vi "nndirectcontrol.vi"() -> ()   [LabVIEW 2017]
doc: "The Clap Sensor sample project implements a clap sensor that detects claps and displays the intensity of the claps by using the onboard LEDs of myRIO."
uses:
  <vilib>/myRIO/Instrument Drivers/Onboard IO/AI/typedefs/AI Reference.ctl
  <vilib>/myRIO/Common/Instrument Driver Framework/Utilities/typedefs/myRIO Generic Hardware Reference.ctl
  <vilib>/myRIO/Common/Instrument Driver Framework/Utilities/typedefs/Hardware Version Enum.ctl
  <vilib>/myRIO/Common/Instrument Driver Framework/Utilities/typedefs/myRIO v1.0 Reference.ctl
  <vilib>/myRIO/Common/Instrument Driver Framework/Utilities/typedefs/Generic FPGA Reference.ctl
  <vilib>/myRIO/Common/Instrument Driver Framework/myRIO v1.0/AI/typedefs/AI Channels List.ctl
  <vilib>/myRIO/Common/Instrument Driver Framework/myRIO v1.0/AI/typedefs/AI Channels Enum.ctl
  <vilib>/myRIO/Common/Instrument Driver Framework/Utilities/typedefs/Analog Scaling Constants List.ctl
  <vilib>/myRIO/Common/Instrument Driver Framework/Utilities/typedefs/Analog Scaling Constants.ctl
  <vilib>/userdefined/High Color/nirio_resource_hc.ctl
  <vilib>/myRIO/Instrument Drivers/Onboard IO/PWM/typedefs/PWM Reference.ctl
  <vilib>/myRIO/Common/Instrument Driver Framework/myRIO v1.0/PWM/typedefs/PWM Channels Enum.ctl
  <vilib>/myRIO/Instrument Drivers/Onboard IO/PWM/typedefs/PWM Configuration.ctl
  <vilib>/myRIO/Common/Instrument Driver Framework/Utilities/vis/Is FPGA Ref Available.vi
  <vilib>/myRIO/Common/Instrument Driver Framework/myRIO v1.0/AI/vis/myRIO v1.1 Open AI.vi
  <vilib>/myRIO/Instrument Drivers/Onboard IO/AI/vis/Read.vi
  <vilib>/myRIO/Common/Instrument Driver Framework/myRIO v1.0/PWM/vis/myRIO v1.1 Open PWM.vi
  <vilib>/myRIO/Instrument Drivers/Onboard IO/PWM/vis/Set Duty Cycle and Frequency.vi
  <vilib>/myRIO/Common/Instrument Driver Framework/Utilities/vis/Validate Channels.vi
  <vilib>/myRIO/Common/Instrument Driver Framework/myRIO v1.0/AI/vis/myRIO v1.0 Reserve AI.vi
  <vilib>/myRIO/Common/Instrument Driver Framework/myRIO v1.0/PWM/vis/myRIO v1.0 Reserve PWM.vi
  <vilib>/myRIO/Common/Instrument Driver Framework/myRIO v1.0/UART/vis/myRIO v1.0 Close UART.vi
  <vilib>/myRIO/Common/Instrument Driver Framework/myRIO v1.0/AI/vis/myRIO v1.0 Build MUX Configuration AI.vi
  <vilib>/myRIO/Common/Instrument Driver Framework/myRIO v1.0/Resource Manager/vis/myRIO v1.0 Reserve Channel List.vi
  <vilib>/myRIO/Common/Instrument Driver Framework/myRIO v1.0/PWM/vis/myRIO v1.0 Build MUX Configuration PWM.vi
  <vilib>/myRIO/Common/Instrument Driver Framework/myRIO v1.0/Resource Manager/vis/myRIO v1.0 Reserve Channel.vi
  <vilib>/myRIO/Common/Instrument Driver Framework/myRIO v1.0/Resource Manager/vis/myRIO v1.0 Unreserve Channel.vi
  <vilib>/myRIO/Common/Instrument Driver Framework/myRIO v1.0/Resource Manager/vis/myRIO v1.0 Create Configuration List.vi
  <vilib>/myRIO/Common/Instrument Driver Framework/myRIO v1.0/Resource Manager/vis/myRIO v1.0 Build Mutex Name.vi
  <vilib>/Utility/VariantDataType/GetNumericInfo.vi
  <vilib>/Utility/error.llb/Error Cluster From Error Code.vi
  <vilib>/myRIO/Common/Instrument Driver Framework/myRIO v1.0/myRIO v1.1 Open.vi
  <vilib>/myRIO/Common/Instrument Driver Framework/myRIO v1.0/AI/vis/myRIO v1.0 Get Scaling Constants AI.vi
  <vilib>/myRIO/Common/Instrument Driver Framework/Utilities/vis/IO Manager.vi
  <vilib>/myRIO/Common/Instrument Driver Framework/Utilities/vis/Configuration Manager.vi
  <vilib>/myRIO/Common/Instrument Driver Framework/myRIO v1.0/myRIO v1.0 Close.vi
  <vilib>/myRIO/Common/Instrument Driver Framework/myRIO v1.0/AI/vis/myRIO v1.0 Read AI.vi
  <vilib>/imath/engines/lvmath2/RunTimeEngine/IndexRead/NIMS M(S,S).vi
  <instcachedir>/0/NIMS M(S,S)_AC51E74150A542F7991B9634C66F3096.lvgen/NIMS M(S,S)_AC51E74150A542F7991B9634C66F3096_000.vi
  <vilib>/imathl/engines/lvmath/Functions/Error Handling/Create Error.vi
  <vilib>/imath/engines/lvmath2/RunTimeEngine/IndexReplace/NIMS V(S)=S.vi
  <instcachedir>/0/NIMS V(S)=S_3F4D177D41884A9C969E5FA0B22E4B28.lvgen/NIMS V(S)=S_3F4D177D41884A9C969E5FA0B22E4B28_000.vi
  <vilib>/imath/engines/lvmath2/RunTimeEngine/IndexRead/NIMS V(S).vi
  <instcachedir>/0/NIMS V(S)_0488751826AF41519A22953C041130DC.lvgen/NIMS V(S)_0488751826AF41519A22953C041130DC_000.vi
  <vilib>/imath/engines/lvmath2/RunTimeEngine/ErrorHandling/NIMS_Create Error From Enums.vi
  <vilib>/imath/engines/lvmath2/RunTimeEngine/IndexReplace/NIMS M(S,S)=S.vi
  <instcachedir>/0/NIMS M(S,S)=S_490F2BBDD0204024B81939EC402D9A55.lvgen/NIMS M(S,S)=S_490F2BBDD0204024B81939EC402D9A55_000.vi
  <vilib>/imath/engines/lvmath2/RunTimeEngine/NodeEndStatement/NIMS_NodeEndStatement_Output.vi
  <instcachedir>/0/NIMS_NodeEndStatement_Output_53EC0D466D134D7ABD903AC30B43404B.lvgen/NIMS_NodeEndStatement_Output_53EC0D466D134D7ABD903AC30B43404B_001.vi
  <instcachedir>/0/NIMS_NodeEndStatement_Output_53EC0D466D134D7ABD903AC30B43404B.lvgen/NIMS_NodeEndStatement_Output_53EC0D466D134D7ABD903AC30B43404B_005.vi
  <instcachedir>/0/NIMS_NodeEndStatement_Output_53EC0D466D134D7ABD903AC30B43404B.lvgen/NIMS_NodeEndStatement_Output_53EC0D466D134D7ABD903AC30B43404B_002.vi
  <vilib>/imath/engines/lvmath2/RunTimeEngine/ErrorHandling/NIMS_Finalize Error.vi
  <vilib>/myRIO/Common/Instrument Driver Framework/myRIO v1.0/Resource Manager/vis/myRIO v1.0 Configure IO.vi
  <vilib>/myRIO/Common/Instrument Driver Framework/myRIO v1.0/PWM/vis/myRIO v1.0 Write PWM.vi
  <vilib>/myRIO/Common/Instrument Driver Framework/Utilities/vis/FPGA Ref Manager.vi
  <vilib>/myRIO/Common/Instrument Driver Framework/myRIO v1.0/myRIO v1.0 Reset FPGA.vi
  <vilib>/myRIO/Common/Instrument Driver Framework/myRIO v1.0/IRQ/vis/myRIO v1.0 IRQ Info FGV.vi
  <vilib>/myRIO/Common/Instrument Driver Framework/myRIO v1.0/IRQ/vis/myRIO v1.0 Timer IRQ Info FGV.vi
  <vilib>/myRIO/Common/Instrument Driver Framework/myRIO v1.0/IRQ/vis/myRIO v1.0 ISR Agent.vi
  <vilib>/myRIO/Express VI/Onboard IO/AI/AI Express VI.xnode
  <vilib>/myRIO/Instrument Drivers/Onboard IO/AI/vis/myRIO AI Open.xnode
  <vilib>/myRIO/Express VI/Onboard IO/PWM/PWM Express VI.xnode
  <vilib>/myRIO/Instrument Drivers/Onboard IO/PWM/vis/myRIO PWM Open.xnode
  <vilib>/myRIO/Instrument Drivers/Utilities/Utilities.lvlib
  <vilib>/myRIO/Instrument Drivers/Onboard IO/AI/AI.lvlib
  <vilib>/myRIO/Instrument Drivers/Onboard IO/PWM/PWM.lvlib
panel:
  in  "step":dbl
  in  "delay":dbl
  in  "max":dbl
  in  "min":dbl
  in  "Staircase":bool
  in  "Sine Ampl.":dbl(slide) scale=0.0..0.5
  in  "Sine freq.":dbl(slide) scale=0.025..0.2
  out "Waveform Chart 2":dbl(graph)
  out "Waveform Chart":cluster{"pa":dbl, "Pdeseada":dbl}(graph)
  out "error [%]":dbl
  in  "PWM [Hz]":dbl=60.0 min=60.0 step=5.0
  out "e1":dbl
  out "eo":dbl
  in  "sample time":u32=20 min=20 step=5
  out "Potentiometer":dbl
  out "yk":dbl
  out "v":dbl[](array[numeric])
  out "w":dbl[][](array[numeric])
  in  "eta":dbl
  in  "Stop":bool
  in  "Pot. (Desired)":dbl=2.0 min=1.6 max=3.6 step=0.2
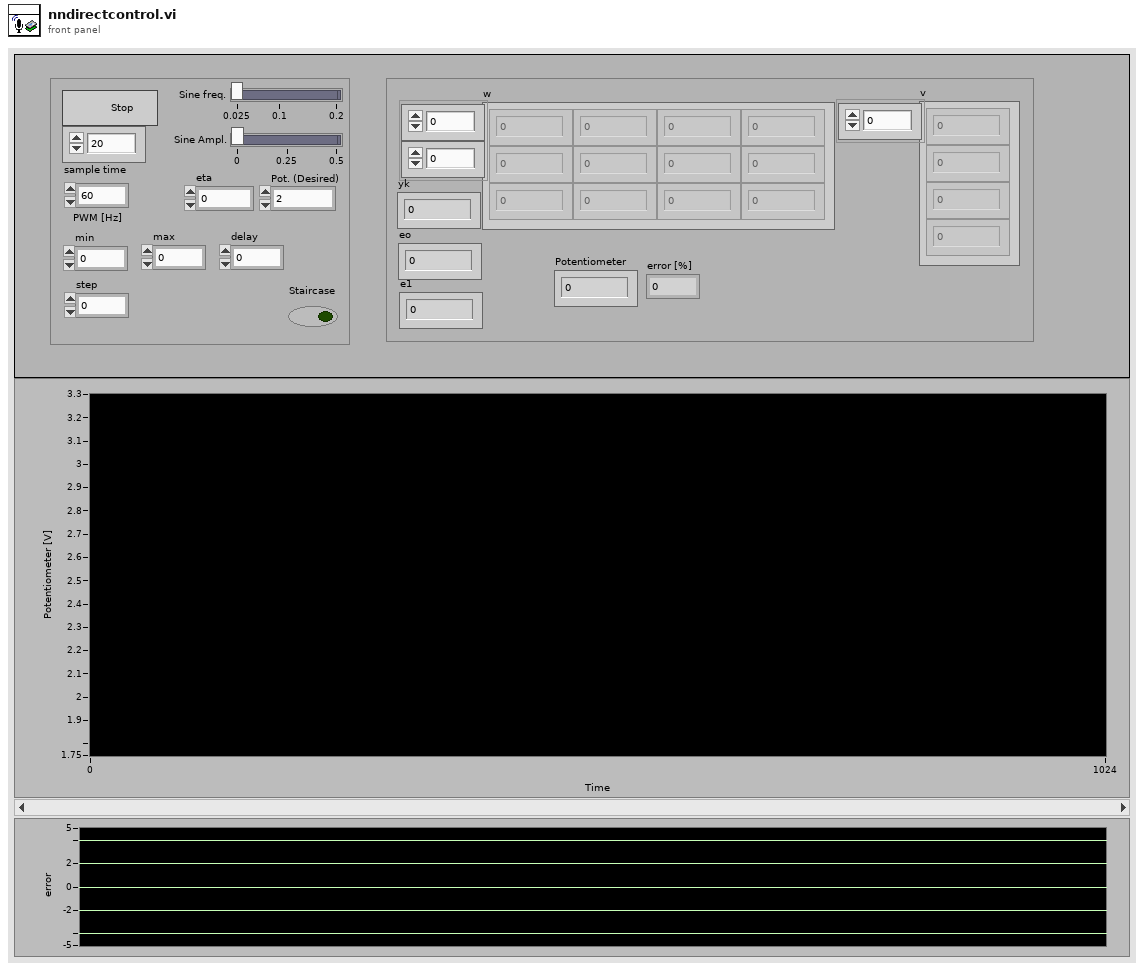
[diagram p1: front panel]
types:
  T1 = typedef "PWM.lvlib/PWM Reference.ctl" = cluster{"myRIO Reference":T2, "PWM Channels Enum":T6, "PWM Configuration":T7}
  T2 = typedef "myRIO Generic Hardware Reference.ctl" = cluster{"myRIO Model":T3, "myRIO Hardware Reference":T4}
  T3 = typedef "Hardware Version Enum.ctl" = enum16{"Unknown", "myRIO-1900", "myRIO-1950", "roboRIO", "NI ELVIS RIO CM"}
  T4 = typedef "myRIO v1.0 Reference.ctl" = cluster{"Generic FPGA Reference":T5, "Allow multiple opens":bool}
  T5 = typedef "Generic FPGA Reference.ctl" = refnum<k20>
  T6 = typedef "PWM Channels Enum.ctl" = enum16{"Not Connected", "C/PWM0", "C/PWM1", "A/PWM0", "A/PWM1", "A/PWM2", "B/PWM0", "B/PWM1", "B/PWM2", "PWM/PWM0", "PWM/PWM1", "PWM/PWM2", "PWM/PWM3", "PWM/PWM4", "PWM/PWM5", "PWM/PWM6", "PWM/PWM7", "PWM/PWM8", "PWM/PWM9"}
  T7 = typedef "PWM.lvlib/PWM Configuration.ctl" = cluster{"Frequency":dbl, "Duty Cycle":dbl}
  T8 = typedef "nirio_resource_hc.ctl" = tag
  T9 = typedef "AI.lvlib/AI Reference.ctl" = cluster{"myRIO Reference":T2, "AI Channels List":T10, "AI Scaling Constants List":T12}
  T10 = typedef "AI Channels List.ctl" = T11[]
  T11 = typedef "AI Channels Enum.ctl" = enum16{"Not Connected", "AudioIn/Left", "AudioIn/Right", "C/AI0", "C/AI1", "A/AI0", "A/AI1", "A/AI2", "A/AI3", "B/AI0", "B/AI1", "B/AI2", "B/AI3", "AI/AI0", "AI/AI1", "AI/AI2", "AI/AI3"}
  T12 = typedef "Analog Scaling Constants List.ctl" = T13[]
  T13 = typedef "Analog Scaling Constants.ctl" = cluster{"LSB Weight (Volts)":dbl, "Offset (Volts)":dbl, "Signed?":bool}
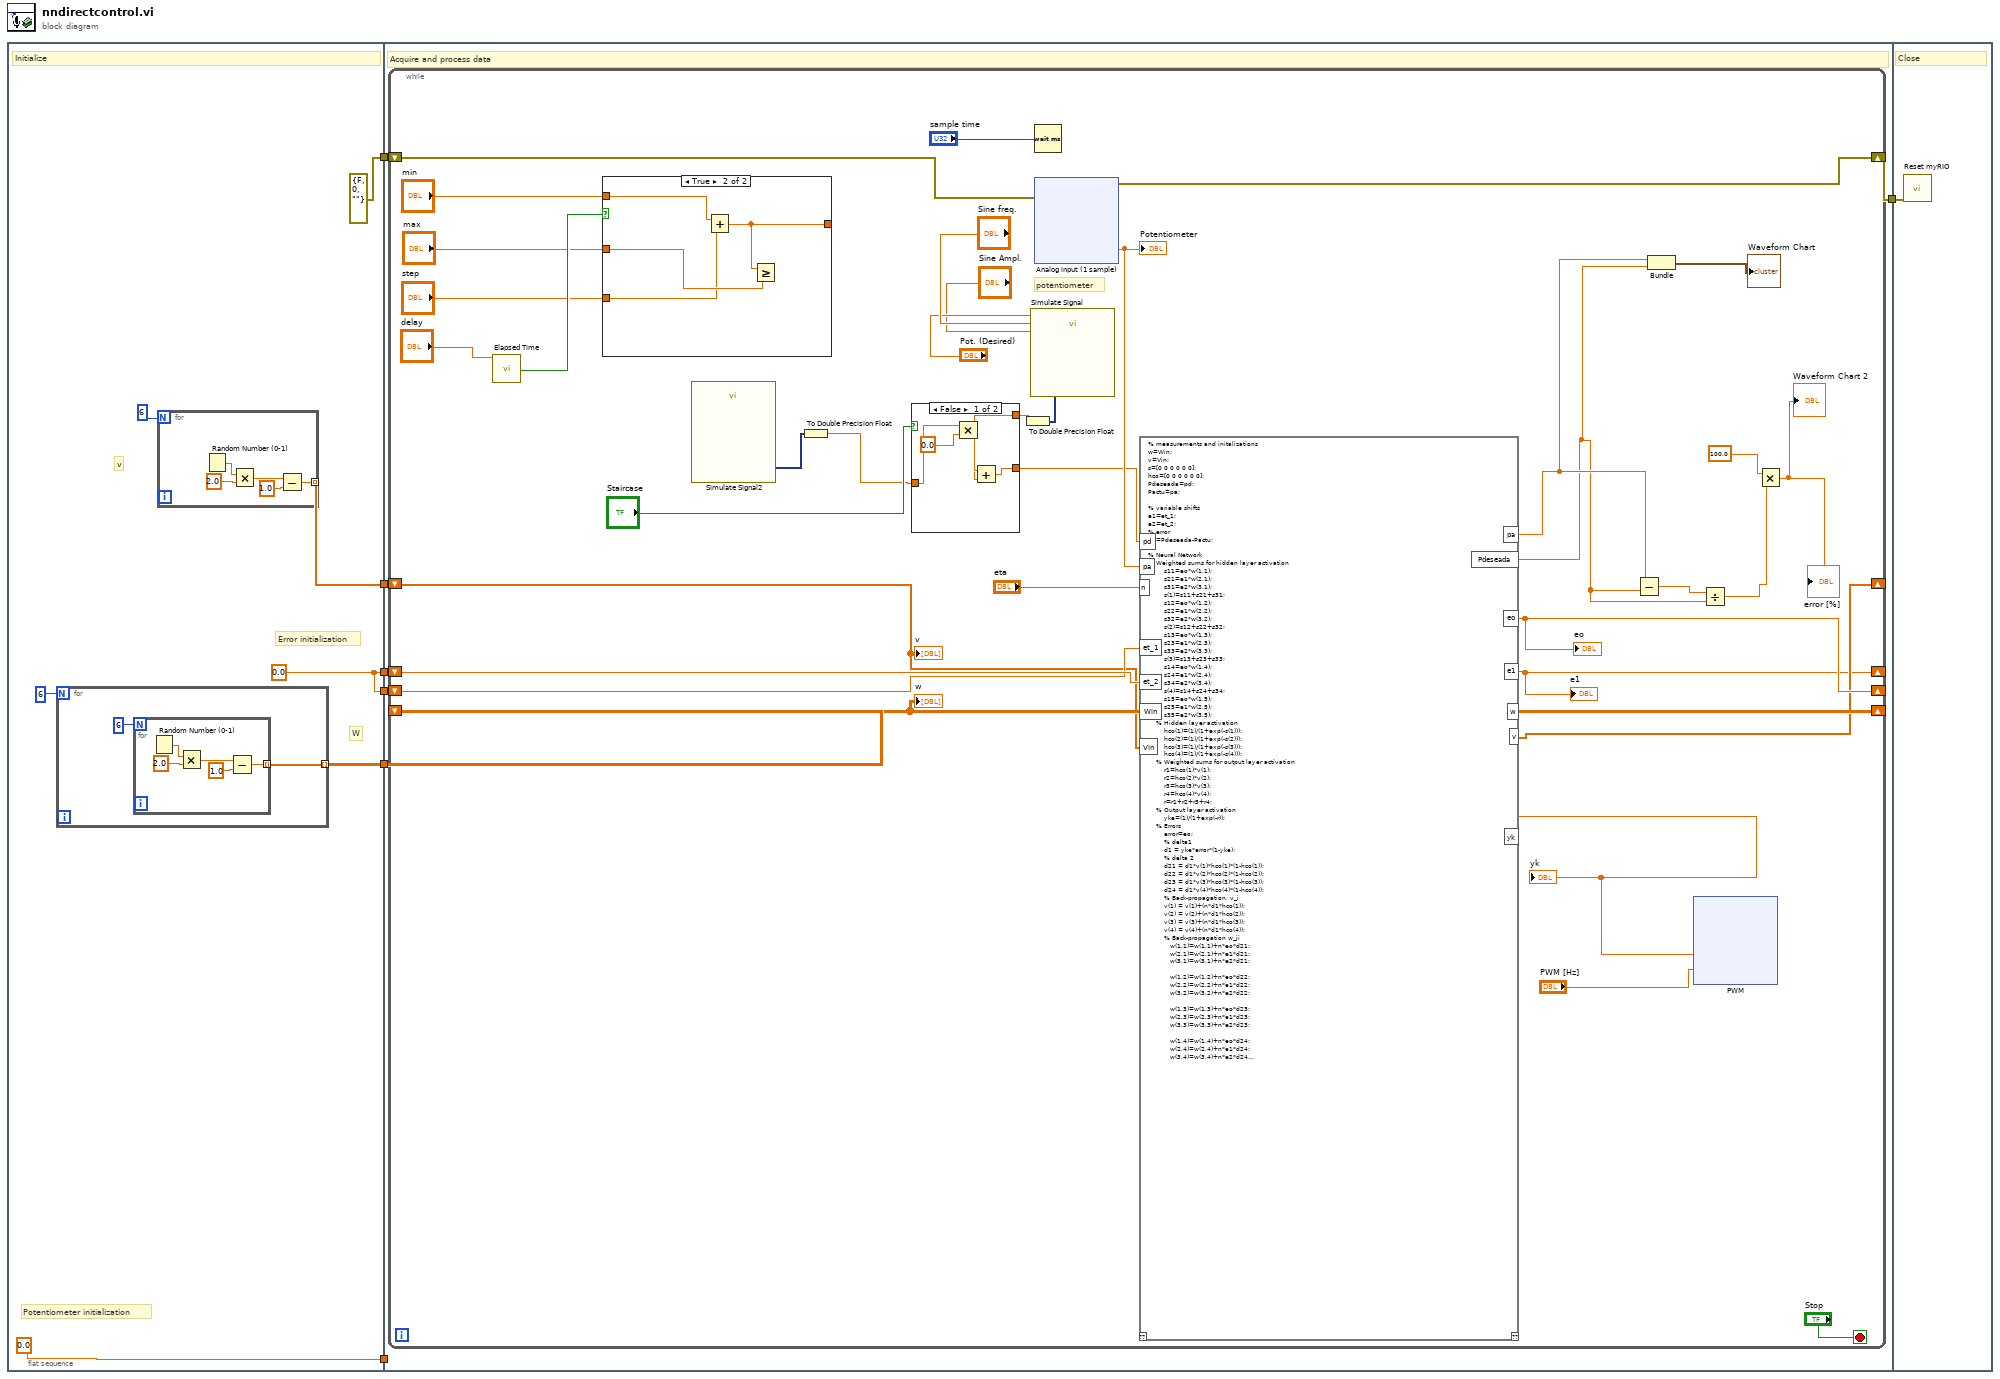
[diagram p0: block diagram]
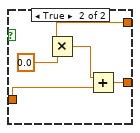
[diagram p3: hidden frame]
diagram:
  n1 = flat-sequence {
    tunnel: [errorcluster {"status"=FALSE, "code"=0, "source"=""} ("error in (no error)")] -> w7
    tunnel: [w13] -> w5
    tunnel: [w13] -> w4
    tunnel: [w11] -> w3
    tunnel: [w9] -> w2
    tunnel: [0.0] -> w1
    tunnel: w7 -> [w32]
    tunnel: [w31] -> w6
    tunnel: w5 -> [w30]
    tunnel: w4 -> [w29]
    tunnel: w3 -> [w28]
    tunnel: w2 -> [w27]
    tunnel: w1 -> [_]
    tunnel: w6 -> [w1645]
    frame #0 {
      w13 = 0.0
      # "Potentiometer initialization"
      # "v"
      # "W"
      # "Error initialization"
      # "Initialize"
      n2 = for {
        N: 6 -> [_]
        tunnel: [w20] -> w11 mode=indexing
        n3 = for {
          N: 6 -> [_]
          tunnel: [w22] -> w20 mode=indexing
          n4 = Random Number (0-1)() -> (number: 0 to 1=w26:dbl)
          n5 = Multiply(x=w26, y=2.0) -> (x*y=w23:dbl)
          n6 = Subtract(x=w23, y=1.0) -> (x-y=w22:dbl)
        }
      }
      n7 = for {
        N: 6 -> [_]
        tunnel: [w15] -> w9 mode=indexing
        n8 = Random Number (0-1)() -> (number: 0 to 1=w19:dbl)
        n9 = Multiply(x=w19, y=2.0) -> (x*y=w16:dbl)
        n10 = Subtract(x=w16, y=1.0) -> (x-y=w15:dbl)
      }
    }
    frame #1 {
      # "Acquire and process data"
      n11 = while {
        shift-right: [w67] -> w31
        shift-left: w32 -> [w68]
        shift-right: [w56] -> _
        shift-left: w30 -> [w65]
        shift-right: [w60] -> _
        shift-left: w29 -> [w64]
        shift-right: [w61] -> _
        shift-left: w28 -> [w63]
        shift-right: [w57] -> _
        shift-left: w27 -> [w62]
        stop <- "Stop" stop-if-true
        # "potentiometer"
        n12 = call "Elapsed Time"("Time Target (s)"="delay") -> ("Time has Elapsed"=w38:bool)  [unwired: 11 in, 7 out]
        n13 = case shown="True" w38 {
          tunnel: "min" -> [w70 w73]
          tunnel: "max" -> [_ w74]
          tunnel: "step" -> [_ w72]
          tunnel: [w70 w71] -> _
          frame False {
          }
          frame True {
            n14 = Add(x=w73, y=w72) -> (x+y=w71:dbl)
            n15 = Greater Or Equal?(x=w71, y=w74) -> ()  [unwired: 1 out]
          }
        }
        n16 = call "Simulate Signal2"() -> ("Triangle"=w34:dynamicdata)  [unwired: 14 in, 1 out]
        n17 = To Double Precision Float(number=w34) -> (double precision float=w33:dbl)
        n18 = call "Simulate Signal"("Offset"="Pot. (Desired)", "Frequency"="Sine freq.", "Amplitude"="Sine Ampl.") -> ("Sine"=w44:dynamicdata)  [unwired: 11 in, 1 out]
        n19 = To Double Precision Float(number=w44) -> (double precision float=w42:dbl)
        n20 = case shown="False" "Staircase" {
          tunnel: w42 -> [w75 w84]
          tunnel: [w77 w82] -> w41
          tunnel: w33 -> [w78 w80]
          frame False {
            n21 = Multiply(x=w78, y=0.0) -> (x*y=w76:dbl)
            n22 = Add(x=w76, y=w75) -> (x+y=w77:dbl)
          }
          frame True {
            n23 = Multiply(x=w84, y=0.0) -> (x*y=w81:dbl)
            n24 = Add(x=w81, y=w80) -> (x+y=w82:dbl)
          }
        }
        n25 = Wait (ms)(milliseconds to wait="sample time") -> ()  [unwired: 1 out]
        n26 = xnode "Analog input (1 sample)"("error in (no error)"=w68) -> ("ENTRADApotenciometro (A/AI3 (Pin 9))"=w59:dbl, "error out"=w67:errorcluster)
        "Potentiometer" <- w59
        n27 = mathscript code="% measurements and initalizations\nw=Win;\nv=Vin;\ns=[0 0 0 0 0 0];\nhco=[0 0 0 0 0 0];\nPdeseada=pd;\nPactu=pa;\n\n% variable shifts\ne1=et_1;\ne2=et_2;\n% error\neo=Pdeseada-Pactu;\n\n% Neural Network\n% Weighted sums for hidden layer activation\n        s11=eo*w(1,1);\n        s21=e1*w(2,1);\n        s31=e2*w(3,1);\n        s(1)=s11+s21+s31;\n        s12=eo*w(1,2);\n        s22=e1*w(2,2);\n        s32=e2*w(3,2);\n        s(2)=s12+s22+s32;\n        s13=eo*w(1,3);\n        s23=e1*w(2,3);\n        s33=e2*w(3,3);\n        s(3)=s13+s23+s33;\n        s14=eo*w(1,4);\n        s24=e1*w(2,4);\n        s34=e2*w(3,4);\n        s(4)=s14+s24+s34;\n        s15=eo*w(1,5);\n        s25=e1*w(2,5);\n        s35=e2*w(3,5);\n    % Hidden layer activation\n        hco(1)=(1)/(1+exp(-s(1)));\n        hco(2)=(1)/(1+exp(-s(2)));\n        hco(3)=(1)/(1+exp(-s(3)));\n        hco(4)=(1)/(1+exp(-s(4)));\n    % Weighted sums for output layer activation\n        r1=hco(1)*v(1);\n        r2=hco(2)*v(2);\n        r3=hco(3)*v(3);\n        r4=hco(4)*v(4);\n        r=r1+r2+r3+r4;\n    % Output layer activation\n        yke=(1)/(1+exp(-r));\n    % Errors\n        error=eo;\n        % delta1\n        d1 = yke*error*(1-yke); \n        % delta 2\n        d21 = d1*v(1)*hco(1)*(1-hco(1));\n        d22 = d1*v(2)*hco(2)*(1-hco(2));\n        d23 = d1*v(3)*hco(3)*(1-hco(3));\n        d24 = d1*v(4)*hco(4)*(1-hco(4));\n        % Back-propagation, v_i\n        v(1) = v(1)+(n*d1*hco(1));\n        v(2) = v(2)+(n*d1*hco(2));\n        v(3) = v(3)+(n*d1*hco(3));\n        v(4) = v(4)+(n*d1*hco(4));\n        % Back-propagation w_ji\n           w(1,1)=w(1,1)+n*eo*d21; \n           w(2,1)=w(2,1)+n*e1*d21;\n           w(3,1)=w(3,1)+n*e2*d21;\n        \n           w(1,2)=w(1,2)+n*eo*d22; \n           w(2,2)=w(2,2)+n*e1*d22;\n           w(3,2)=w(3,2)+n*e2*d22;\n           \n           w(1,3)=w(1,3)+n*eo*d23; \n           w(2,3)=w(2,3)+n*e1*d23;\n           w(3,3)=w(3,3)+n*e2*d23;\n           \n           w(1,4)=w(1,4)+n*eo*d24; \n           w(2,4)=w(2,4)+n*e1*d24;\n           w(3,4)=w(3,4)+n*e2*d24;\n        \nyk = yke;"("pa"=w59, "n"="eta", "pd"=w41, "et_1"=w64, "et_2"=w65, "Win"=w63, "Vin"=w62) -> ("w"=w61:dbl[][], "eo"=w60:dbl, "yk"=w55:dbl, "v"=w57:dbl[], "e1"=w56:dbl, "pa"=w50:dbl, "Pdeseada"=w49:dbl)  [unwired: 1 in, 1 out]
        "yk" <- w55
        "eo" <- w60
        "e1" <- w56
        n28 = Subtract(x=w50, y=w49) -> (x-y=w53:dbl)
        n29 = Bundle("pa"=w50, "Pdeseada"=w49) -> (→"Waveform Chart":cluster{"pa":dbl, "Pdeseada":dbl})  [unwired: 1 in]
        n30 = xnode "PWM"("Duty Cycle"=w55, "Frequency [Hz]"="PWM [Hz]") -> ()  [unwired: 1 in, 1 out]
        n31 = Divide(x=w53, y=w49) -> (x/y=w52:dbl)
        n32 = Multiply(x=100.0, y=w52) -> (x*y=→"error [%]" →"Waveform Chart 2":dbl)
        "w" <- w63
        "v" <- w62
      }
    }
    frame #2 {
      # "Close"
      n33 = call <vilib>:"Reset myRIO.vi"("error in (no error)"=w1645) -> ()  [unwired: 10 in, 1 out]
    }
  }
